vi "amplitude_modulation_test.vi"() -> ()   [LabVIEW 2017]
uses:
  <userlib>/niRF/niQuickSyn/Core/Properties/VISA Handle/PropertyType.ctl
  <userlib>/niRF/niQuickSyn/Core/Properties/RF Frequency/PropertyType.ctl
  <userlib>/niRF/niQuickSyn/Core/Properties/RF Power/PropertyType.ctl
  <userlib>/niRF/niQuickSyn/Core/Properties/FM Sensitivity/PropertyType.ctl
  <userlib>/niRF/niQuickSyn/Core/Properties/AM State/PropertyType.ctl
  <vilib>/Utility/error.llb/DialogType.ctl
  <userlib>/niRF/niQuickSyn/Core/Properties/RF Output/PropertyType.ctl
  <vilib>/DAQmx/read.llb/DAQmx Read (Analog 1D DBL 1Chan NSamp).vi
  <vilib>/DAQmx/create/channels.llb/DAQmx Create Channel (AI-Voltage-Basic).vi
  <vilib>/DAQmx/configure/timing.llb/DAQmx Timing (Sample Clock).vi
  <vilib>/DAQmx/configure/trigger.llb/DAQmx Start Trigger (None).vi
  <vilib>/DAQmx/miscellaneous.llb/DAQmx Fill In Error Info.vi
  <userlib>/niRF/niQuickSyn/QuickSyn API.lvlib
  <userlib>/niRF/niQuickSyn/Core/Properties/RF Output/RF Output.lvclass
  <resource>/objmgr/daqmx.rc
  <userlib>/niRF/niQuickSyn/Core/Properties/RF Frequency/RF Frequency.lvclass
  <userlib>/niRF/niQuickSyn/Core/Properties/VISA Handle/VISA Handle.lvclass
  <userlib>/niRF/niQuickSyn/Core/Properties/RF Power/RF Power.lvclass
  <userlib>/niRF/niQuickSyn/Core/Properties/FM Sensitivity/FM Sensitivity.lvclass
  <userlib>/niRF/niQuickSyn/Core/Properties/AM State/AM State.lvclass
panel:
  in  "Amplitude":dbl=1.0 min=-2.0 max=2.0
  in  "Frequency":dbl=5000.0
  in  "AM State":T1
  in  "RF Output":bool
  in  "ms to wait":u32=100
  out "error out":errorcluster
  in  "stop":bool
  out "SpectrumGraph":cluster{i32[], dbl[]}(graph)
  out "AI.Max 2":dbl=0.5
  out "AI.Min 2":dbl=-0.5
  in  "AI.Max":dbl=0.5
  in  "samples per channel":i32=500000
  in  "rate":dbl=100000.0 format="%0.0f"
  in  "DAQ channel (in)":tag="DAQ6363/ai1"
  in  "AM Depth":T2 format="%#_9p"
  in  "RF Power, dB (0)":T3 min=-10.0 max=13.0 step=0.1
  in  "RF Frequency":T4=200000000.0 min=500000000.0 max=20000000000.0 step=0.001 format="%#_9p"
  in  "error in (no error)":errorcluster
  in  "QuickSyn Name (in)":T5="COM5"
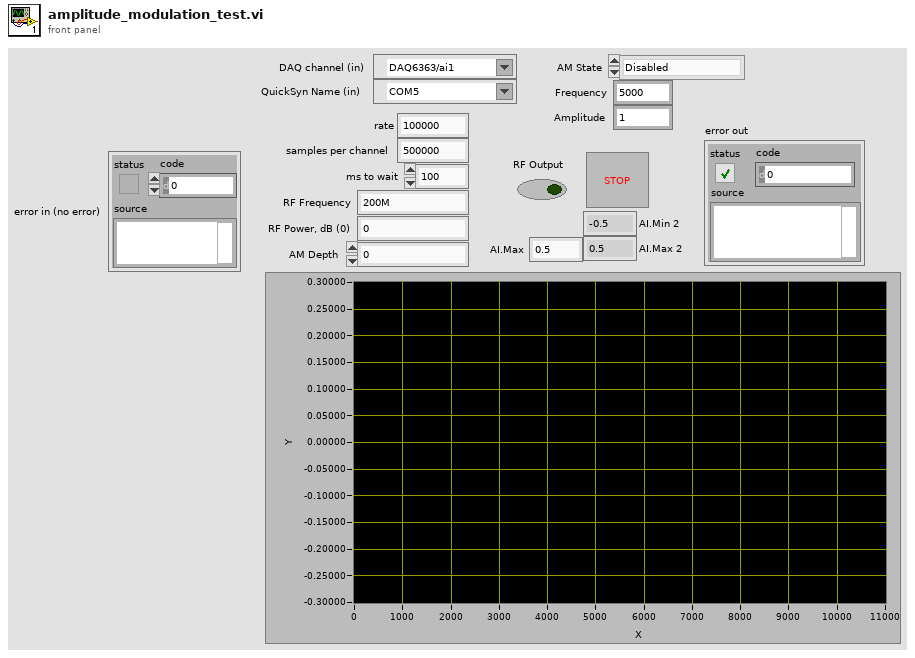
[diagram p1: front panel]
types:
  T1 = typedef "QuickSyn API.lvlib/AM State.lvclass/PropertyType.ctl" = enum16{"Disabled", "Enabled"}
  T2 = typedef "QuickSyn API.lvlib/FM Sensitivity.lvclass/PropertyType.ctl" = dbl
  T3 = typedef "QuickSyn API.lvlib/RF Power.lvclass/PropertyType.ctl" = dbl
  T4 = typedef "QuickSyn API.lvlib/RF Frequency.lvclass/PropertyType.ctl" = dbl
  T5 = typedef "QuickSyn API.lvlib/VISA Handle.lvclass/PropertyType.ctl" = refnum<visa-resource-name>
  T6 = typedef "QuickSyn API.lvlib/RF Output.lvclass/PropertyType.ctl" = bool
  T7 = typedef "DialogType.ctl" = u16
  T8 = typedef "QuickSyn API.lvlib/QuickSyn.lvclass/Session Handle.ctl" = refnum<data-value>
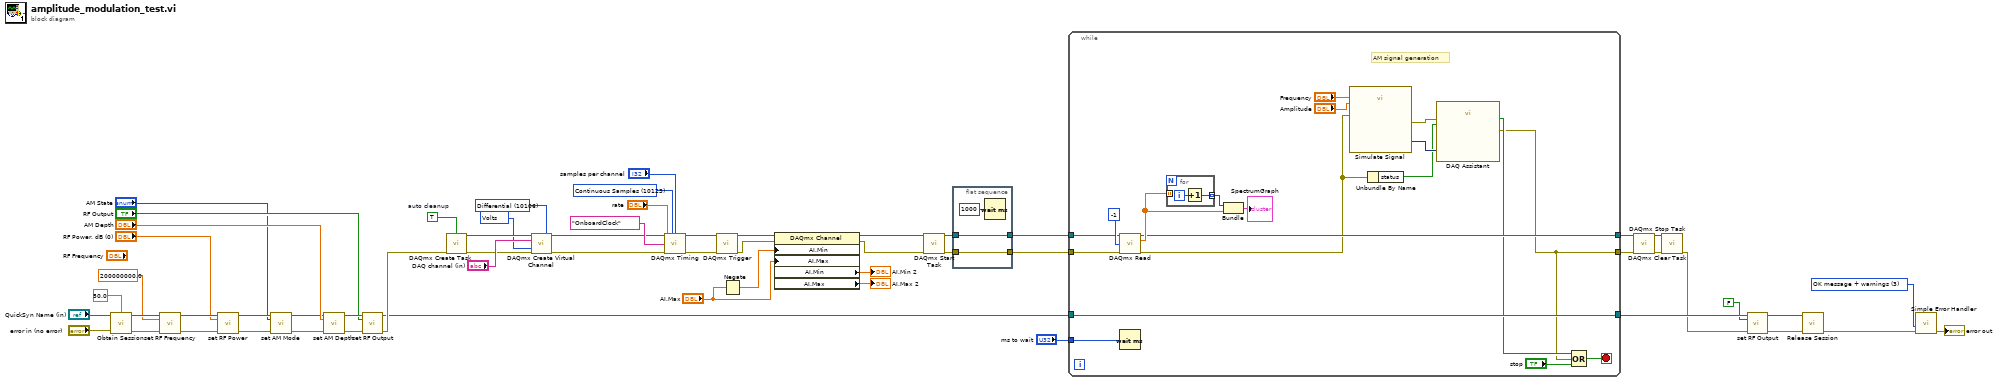
[diagram p0: block diagram]
diagram:
  w17 = T7 3 items=["no dialog", "OK message", "continue or stop message", "OK message + warnings", "continue/stop + warnings"] ("type of dialog (OK msg:1)")
  w41 = TRUE  # auto cleanup
  w43 = 10123 items=["Finite Samples"=10178, "Continuous Samples"=10123, "Hardware Timed Single Point"=12522] ("sample mode")
  w34 = 10106 items=["Default"=-1, "RSE"=10083, "NRSE"=10078, "Differential"=10106, "Pseudodifferential"=12529] ("input terminal configuration")
  w33 = 10348 items=["Volts"=10348, "From Custom Scale"=10065] ("units")
  n1 = call <userlib>:"Obtain Session.vi"("VISA resource name"="QuickSyn Name (in)", "Serial Timeout"=50.0, "error in (no error)"="error in (no error)") -> ("Session Handle"=w53:T8, "error out"=w52:errorcluster)  [unwired: 11 in]
  n2 = call <userlib>:"set RF Frequency.vi"("Session Handle in"=w53, "RF Frequency, Hz (200M)"=T4 200000000.0, "error in (no error)"=w52) -> ("Session Handle out"=w55:T8, "error out"=w56:errorcluster)  [unwired: 11 in]
  n3 = call <userlib>:"set RF Power.vi"("Session Handle in"=w55, "RF Power, dB (0)"="RF Power, dB (0)", "error in (no error)"=w56) -> ("Session Handle out"=w50:T8, "error out"=w51:errorcluster)  [unwired: 11 in]
  n4 = call <userlib>:"set AM Mode.vi"("Session Handle in"=w50, "AM State"="AM State", "error in (no error)"=w51) -> ("Session Handle out"=w48:T8, "error out"=w47:errorcluster)  [unwired: 11 in]
  n5 = call <userlib>:"set AM Depth.vi"("Session Handle in"=w48, "AM Depth"="AM Depth", "error in (no error)"=w47) -> ("Session Handle out"=w46:T8, "error out"=w45:errorcluster)  [unwired: 11 in]
  n6 = call <userlib>:"set RF Output.vi"("Session Handle in"=w46, "RF Output (False)"="RF Output", "error in (no error)"=w45) -> ("Session Handle out"=w25:T8, "error out"=w28:errorcluster)  [unwired: 11 in]
  n7 = call <vilib>:"DAQmx Create Task.vi"("auto cleanup"=w41, "error in"=w28) -> ("task out"=w40:refnum<k21>, "error out"=w39:errorcluster)  [unwired: 12 in]
  n8 = call-poly <vilib>:"DAQmx Create Virtual Channel.vi"("task in"=w40, "input terminal configuration"=w34, "physical channels"="DAQ channel (in)", "units"=w33, "error in"=w39) -> ("task out"=w32:refnum<k21>, "error out"=w31:errorcluster)  [unwired: 9 in]
  n9 = call-poly <vilib>:"DAQmx Timing.vi"("task/channels in"=w32, "sample mode"=w43, "samples per channel"="samples per channel", "rate"="rate", "source"=tag "OnboardClock", "error in"=w31) -> ("task out"=w38:refnum<k21>, "error out"=w37:errorcluster)  [unwired: 8 in]
  n10 = call-poly <vilib>:"DAQmx Trigger.vi"("task/channels in"=w38, "error in"=w37) -> ("task out"=w30:refnum<k21>, "error out"=w29:errorcluster)  [unwired: 12 in]
  n11 = Negate(x="AI.Max") -> (-x=w1:dbl)
  n12 = property class="DAQmx Channel"(reference=w30, error in=w29, "AI.Min"=w1, "AI.Max"="AI.Max") -> (reference out=w22:refnum<k21>, error out=w21:errorcluster, "AI.Min"=→"AI.Min 2":dbl, "AI.Max"=→"AI.Max 2":dbl)
  n13 = call <vilib>:"DAQmx Start Task.vi"("task/channels in"=w22, "error in"=w21) -> ("task out"=w24:refnum<k21>, "error out"=w23:errorcluster)  [unwired: 12 in]
  n14 = flat-sequence {
    tunnel: w23 -> [w62]
    tunnel: [w62] -> w19
    tunnel: w24 -> [w61]
    tunnel: [w61] -> w20
    frame #0 {
      n15 = Wait (ms)(milliseconds to wait=u32 1000) -> ()  [unwired: 1 out]
    }
  }
  n16 = while {
    tunnel: w25 -> [w75]
    tunnel: w20 -> [w80]
    tunnel: w19 -> [w79]
    tunnel: [w71] -> w14
    tunnel: [w75] -> w10
    tunnel: [w74] -> w13
    tunnel: "ms to wait" -> [w73]
    stop <- w69 stop-if-true
    # "AM signal generation"
    n17 = call-poly <vilib>:"DAQmx Read.vi"("task/channels in"=w80, "number of samples per channel"=-1, "error in"=w79) -> ("task out"=w74:refnum<k21>, "data"=w76:dbl[], "error out"=w64:errorcluster)  [unwired: 10 in]
    n18 = Wait (ms)(milliseconds to wait=w73) -> ()  [unwired: 1 out]
    n19 = for {
      tunnel: [w82] -> w78 mode=indexing
      tunnel: w76 -> [_] mode=indexing
      i -> [w83]
      n20 = Increment(x=w83) -> (x+1=w82:i32)
    }
    n21 = Bundle(w78, "data"=w76) -> (→"SpectrumGraph":cluster{i32[], "data":dbl[]})  [unwired: 1 in]
    n22 = call "Simulate Signal"("Frequency"="Frequency", "Amplitude"="Amplitude", "error in (no error)"=w64) -> ("Sine"=w65:dynamicdata, "error out"=w66:errorcluster)  [unwired: 11 in]
    n23 = Unbundle By Name(w64) -> ("status"=w63:bool)
    n24 = call "DAQ Assistant"("data"=w65, "error in"=w66, "stop (F)"=w63) -> ("stopped"=w72:bool, "error out"=w71:errorcluster)  [unwired: 14 in, 1 out]
    n25 = Compound Arithmetic op=OR(w72, w71, "stop") -> (w69:bool)
  }
  n26 = call <vilib>:"DAQmx Stop Task.vi"("task/channels in"=w13, "error in"=w14) -> ("task out"=w15:refnum<k21>, "error out"=w16:errorcluster)  [unwired: 12 in]
  n27 = call <vilib>:"DAQmx Clear Task.vi"("task in"=w15, "error in"=w16) -> ("error out"=w7:errorcluster)  [unwired: 13 in]
  n28 = call <userlib>:"set RF Output.vi"("Session Handle in"=w10, "RF Output (False)"=T6 FALSE, "error in (no error)"=w7) -> ("Session Handle out"=w9:T8, "error out"=w8:errorcluster)  [unwired: 11 in]
  n29 = call <userlib>:"Release Session.vi"("Session Handle"=w9, "error in (no error)"=w8) -> ("error out"=w12:errorcluster)  [unwired: 13 in]
  n30 = call <vilib>:"Simple Error Handler.vi"("type of dialog (OK msg:1)"=w17, "error in (no error)"=w12) -> ("error out"=→"error out":errorcluster)  [unwired: 3 in, 4 out]
